vi "状态栏-信息生成.vi"(8 "消息内容":string, 11 "消息类型":string) -> (3 "状态消息":string caption="结果")   [LabVIEW 2017]
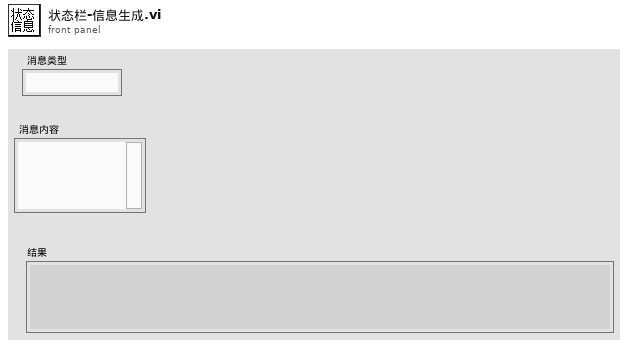
[diagram p1: front panel]
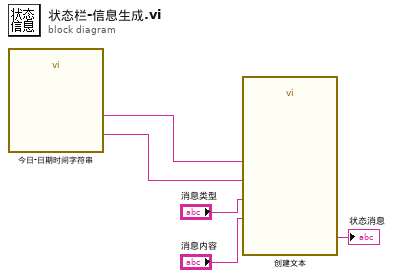
[diagram p0: block diagram]
diagram:
  n1 = call "今日-日期时间字符串.vi"() -> ("hh:mm:ss"=w2:string, "YYYY-MM-DD"=w1:string)  [unwired: 9 in, 1 out]
  n2 = call "创建文本"("消息内容"="消息内容", "日期"=w1, "时间"=w2, "消息类型"="消息类型") -> ("Result"=→"状态消息":string)  [unwired: 10 in, 1 out]
